vi "Tool_Extract and Save First Frame.vi"() -> ()   [LabVIEW 2012]
uses:
  ND2_Reader_32bit/ND2_Reader_32.lvlib
panel:
  out "of":i32
  out "File":i32
  out "N Directories in Queue":i32
  out "Current Directory":path
  in  "Start Processing":bool
  in  "Exit":bool
  in  "Show Hide Image":bool
  in  "Process:":T1(ring)
  in  "Path to .tif file storage":path
  out "Image":T2(plugin-control)
  out "TIFF File":path
  out "ND2 File":path
  in  "Path to ND2 Directories":path
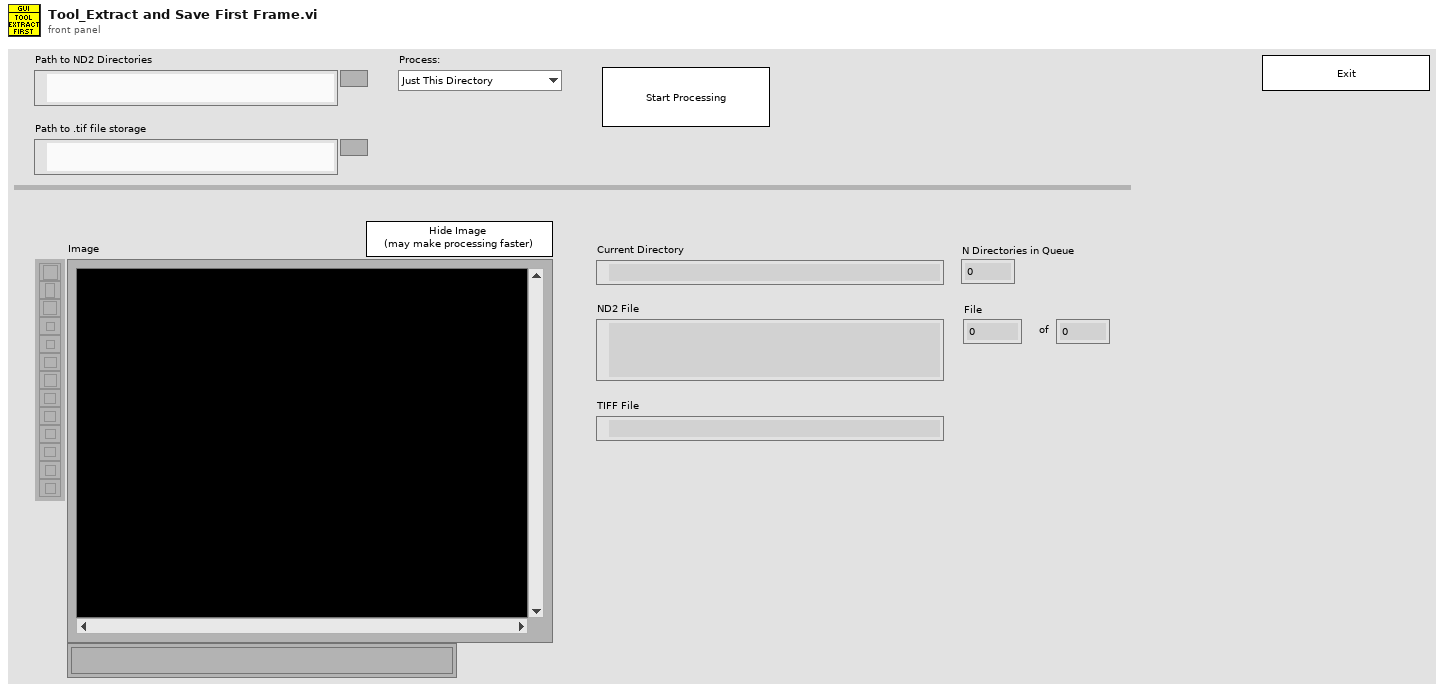
[diagram p1: front panel]
types:
  T1 = enum16{"Just This Directory", "All Sub Directories"}
  T2 = typedef "IMAQ Image.ctl" = refnum<image>
  T3 = typedef "Image Type" = u32
  T4 = typedef "cluster_LIMPICTURE.ctl" = cluster{"uiWidth":u32, "uiHeight":u32, "uiBitsPerComp":u32, "uiComponents":u32, "uiWidthBytes":u32, "uiSize":u32, "pImageData":u32}
  T5 = typedef "numeric_LIMFILEHANDLE.ctl" = i32
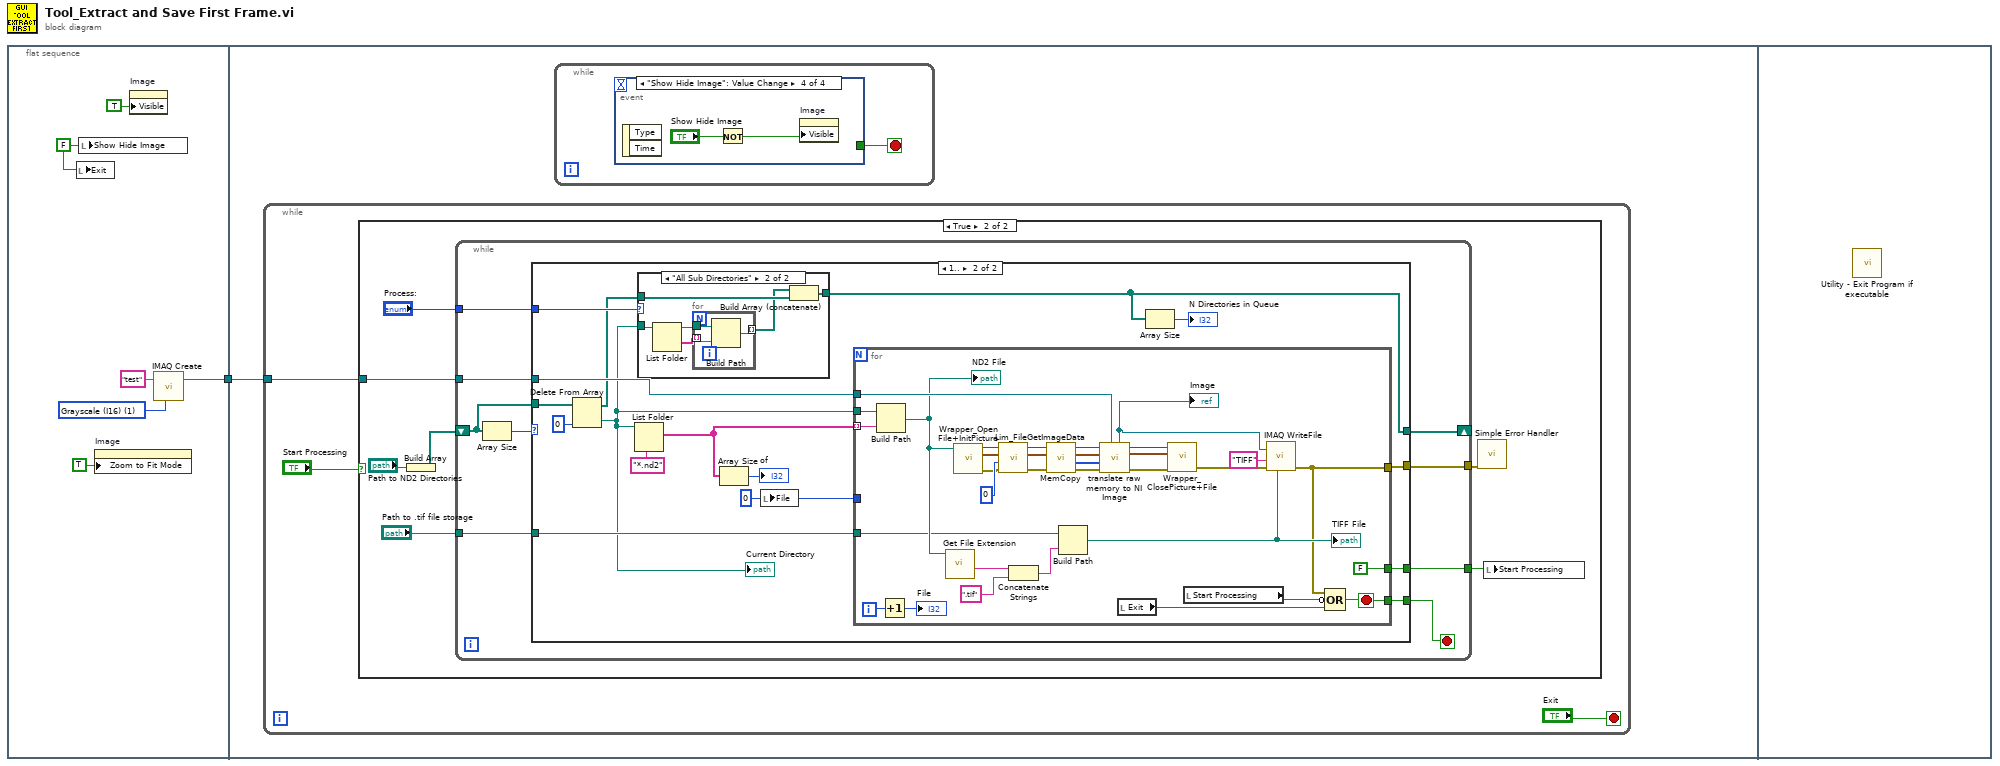
[diagram p0: block diagram]
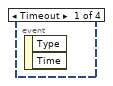
[diagram p2: hidden frame]
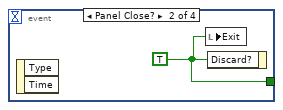
[diagram p3: hidden frame]
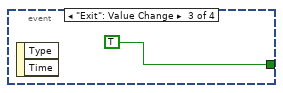
[diagram p4: hidden frame]
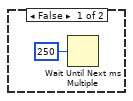
[diagram p5: hidden frame]
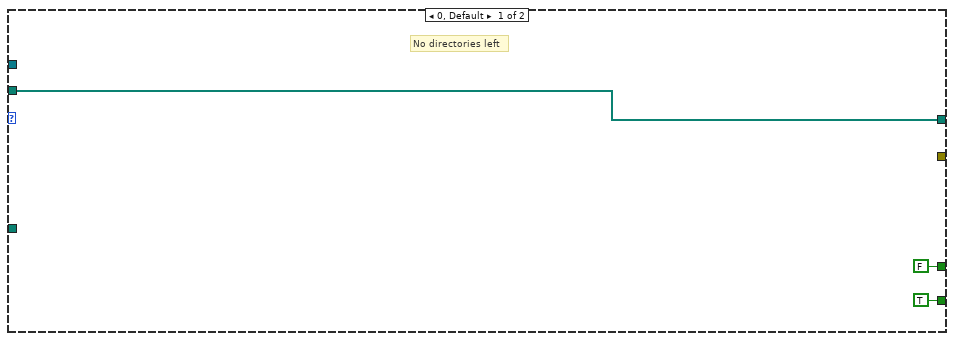
[diagram p6: hidden frame]
diagram:
  n1 = flat-sequence {
    tunnel: [w3] -> w1
    tunnel: w1 -> [w8]
    frame #0 {
      w5 = T3 1 items=["Grayscale (U8)", "Grayscale (I16)", "Grayscale (SGL)", "Complex (CSG)", "RGB (U32)", "HSL (U32)", "RGB (U64)", "Grayscale (U16)"] ("Image Type")
      w6 = FALSE ("Show Hide Image")
      n2 = local write "Exit"(w6) -> ()
      n3 = local write "Show Hide Image"(w6) -> ()
      n4 = property on="Image" class="ImageControl"("Zoom to Fit Mode"=TRUE) -> ()  [unwired: 2 in, 2 out]
      n5 = property on="Image" class="ImageControl"("Visible"=TRUE) -> ()  [unwired: 2 in, 2 out]
      n6 = call "IMAQ Create"("Image Name"="test", "Image Type"=w5) -> ("New Image"=w3:T2)  [unwired: 3 in, 1 out]
    }
    frame #1 {
      n7 = while {
        tunnel: w8 -> [w15]
        stop <- "Exit" stop-if-true
        n8 = case shown="True" "Start Processing" {
          tunnel: w15 -> [_ w21]
          frame False {
            n9 = Wait Until Next ms Multiple(millisecond multiple=u32 250) -> ()  [unwired: 1 out]
          }
          frame True {
            n10 = Build Array("Path to ND2 Directories") -> (w19:path[])
            n11 = while {
              tunnel: [w33] -> w24
              tunnel: "Path to .tif file storage" -> [w32]
              tunnel: [w31] -> w22
              tunnel: w21 -> [w30]
              shift-right: [w26] -> _
              shift-left: w19 -> [w27]
              tunnel: "Process:" -> [w25]
              stop <- w29 stop-if-true
              n12 = Array Size(array=w27) -> (size(s)=w28:i32)
              n13 = case shown="1.." w28 {
                tunnel: [_ w51] -> w33
                tunnel: w32 -> [_ w50]
                tunnel: [FALSE w49] -> w31
                tunnel: w30 -> [_ w48]
                tunnel: [TRUE w47] -> w29
                tunnel: w27 -> [w36 w45]
                tunnel: [w36 w40] -> w26
                tunnel: w25 -> [_ w44]
                frame 0, Default {
                  # "No directories left"
                }
                frame 1.. {
                  w37 = 0 ("File")
                  n14 = Delete From Array(array=w45, index=0) -> (deleted portion=w42:path, array with subset deleted=w43:path[])  [unwired: 1 in]
                  "Current Directory" <- w42
                  n15 = List Folder(path=w42, pattern="*.nd2") -> (filenames=w39:string[])  [unwired: 2 in, 3 out]
                  n16 = case shown="\"All Sub Directories\"" w44 {
                    tunnel: w43 -> [w53 w59]
                    tunnel: [w53 w57] -> w40
                    tunnel: w42 -> [_ w56]
                    frame "Just This Directory" {
                    }
                    frame "All Sub Directories" {
                      n17 = List Folder(path=w56) -> (path out=w55:path, folder names=w54:string[])  [unwired: 3 in, 2 out]
                      n18 = for {
                        tunnel: w54 -> [w60] mode=indexing
                        tunnel: [w62] -> w58 mode=indexing
                        tunnel: w55 -> [w61]
                        n19 = Build Path(base path=w61, name or relative path=w60) -> (appended path=w62:path)
                      }
                      n20 = Build Array (concatenate)(w58, w59) -> (w57:path[])
                    }
                  }
                  n21 = Array Size(array=w39) -> (size(s)=→"of":i32)
                  n22 = local write "File"(w37) -> ()
                  n23 = for {
                    tunnel: w48 -> [w85]
                    tunnel: [w69] -> w51
                    tunnel: w42 -> [w74]
                    tunnel: w39 -> [w81] mode=indexing
                    tunnel: w50 -> [w70]
                    tunnel: [FALSE] -> w49
                    tunnel: [w65] -> w47
                    tunnel: w37 -> [_]
                    i -> [w64]
                    stop <- w65 stop-if-true
                    n24 = Build Path(base path=w74, name or relative path=w81) -> (appended path=w73:path)
                    "ND2 File" <- w73
                    n25 = Increment(x=w64) -> (x+1=→"File":i32)
                    n26 = call <vilib>:"Get File Extension.vi"("file"=w73) -> ("filename without extension"=w77:string)  [unwired: 7 in, 3 out]
                    n27 = call "Wrapper_Open File+InitPicture.vi"("FilePath"=w73) -> ("error out"=w71:errorcluster, "LIMPICTURE"=w79:T4, "hFile out"=w80:T5)  [unwired: 7 in, 1 out]
                    n28 = call "Lim_FileGetImageData.vi"("error in (no error)"=w71, "frameindex"=0, "LIMPICTURE in"=w79, "hFile in"=w80) -> ("error out"=w88:errorcluster, "LIMPICTURE out"=w94:T4, "hFile out"=w95:T5)  [unwired: 4 in, 1 out]
                    n29 = Concatenate Strings(w77, ".tif" ("string")) -> (w75:string)
                    n30 = call "MemCopy.vi"("error in (no error)"=w88, "LIMPICTURE in"=w94, "hFile in"=w95) -> ("error out"=w87:errorcluster, "pBuffer out"=w89:u8[], "LIMPICTURE out"=w92:T4, "hFile out"=w93:T5)  [unwired: 5 in]
                    n31 = Build Path(base path=w70, name or relative path=w75) -> (appended path=w72:path)
                    "TIFF File" <- w72
                    n32 = call "translate raw memory to NI Image.vi"("Image in"=w85, "error in (no error)"=w87, "pBuffer"=w89, "LIMPICTURE in"=w92, "hFile in"=w93) -> ("error out"=w86:errorcluster, "LIMPICTURE out"=w90:T4, "hFile out"=w91:T5, "Image out"=w83:T2)  [unwired: 3 in]
                    "Image" <- w83
                    n33 = local read "Exit"() -> (w67:bool)
                    n34 = call "Wrapper_ClosePicture+File.vi"("error in (no error)"=w86, "LIMPICTURE"=w90, "hFile in"=w91) -> ("error out"=w82:errorcluster)  [unwired: 8 in]
                    n35 = local read "Start Processing"() -> (w68:bool)
                    n36 = call "IMAQ WriteFile"("error in (no error)"=w82, "File Type"="TIFF", "File Path"=w72, "Image"=w83) -> ("error out"=w69:errorcluster)  [unwired: 4 in]
                    n37 = Compound Arithmetic op=OR(w69, invert w68, w67) -> (w65:bool)
                  }
                  n38 = Array Size(array=w40) -> (size(s)=→"N Directories in Queue":i32)
                }
              }
            }
            n39 = call <vilib>:"Simple Error Handler.vi"("error in (no error)"=w24) -> ()  [unwired: 4 in, 5 out]
            n40 = local write "Start Processing"(w22) -> ()
          }
        }
      }
      n41 = while {
        stop <- w9 stop-if-true
        n42 = event shown="[3] \"Show Hide Image\": Value Change" {
          selector: _ -> [_ _ _ _]
          dyn-events: _ -> [_ _ _ _]
          timeout: _ -> [_ _ _ _]
          tunnel: [_ w10 TRUE ("Discard?") _] -> w9
          event Timeout {
            n43 = event-data() -> ()  [unwired: 1 in, 2 out]
          }
          event Panel Close? {
            w10 = TRUE ("Discard?")
            n44 = event-data() -> ()  [unwired: 1 in, 2 out]
            n45 = local write "Exit"(w10) -> ()
            n46 = event-data("Discard?"=w10) -> ()  [unwired: 1 in, 1 out]
          }
          event "Exit": Value Change {
            n47 = event-data() -> ()  [unwired: 1 in, 2 out]
          }
          event "Show Hide Image": Value Change {
            n48 = event-data() -> ()  [unwired: 1 in, 2 out]
            n49 = Not(x="Show Hide Image") -> (.not. x?=w13:bool)
            n50 = property on="Image" class="ImageControl"("Visible"=w13) -> ()  [unwired: 2 in, 2 out]
          }
        }
      }
    }
    frame #2 {
      n51 = call "Utility - Exit Program if executable.vi"() -> ()  [unwired: 11 in, 1 out]
    }
  }
